vi "trim_string_of_wspaces_and_quotes.vi"(3 "Trim whitespaces (Trim both)":u16(ring) items=["Trim both", "Trim start", "Trim end", "Trim none"], 4 "String in":string, 5 "Remove quotes (Remove All)":u16(ring) items=["Remove All Quotes", "Remove Single Quotes", "Remove Double Quotes", "Remove None"]) -> (1 "String out":string)   [LabVIEW 2020, in "Rohde&Schwarz RTx Oscilloscopes.lvlib" / "rsidr_core.lvlib"]
uses:
  rsidr_core.lvlib
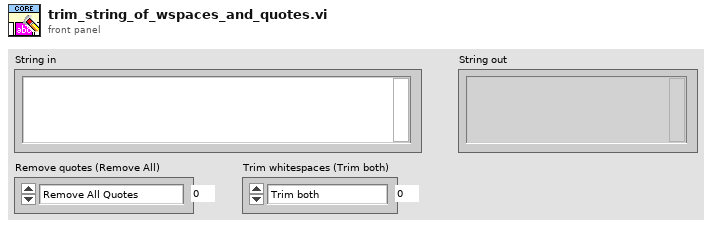
[diagram p1: front panel]
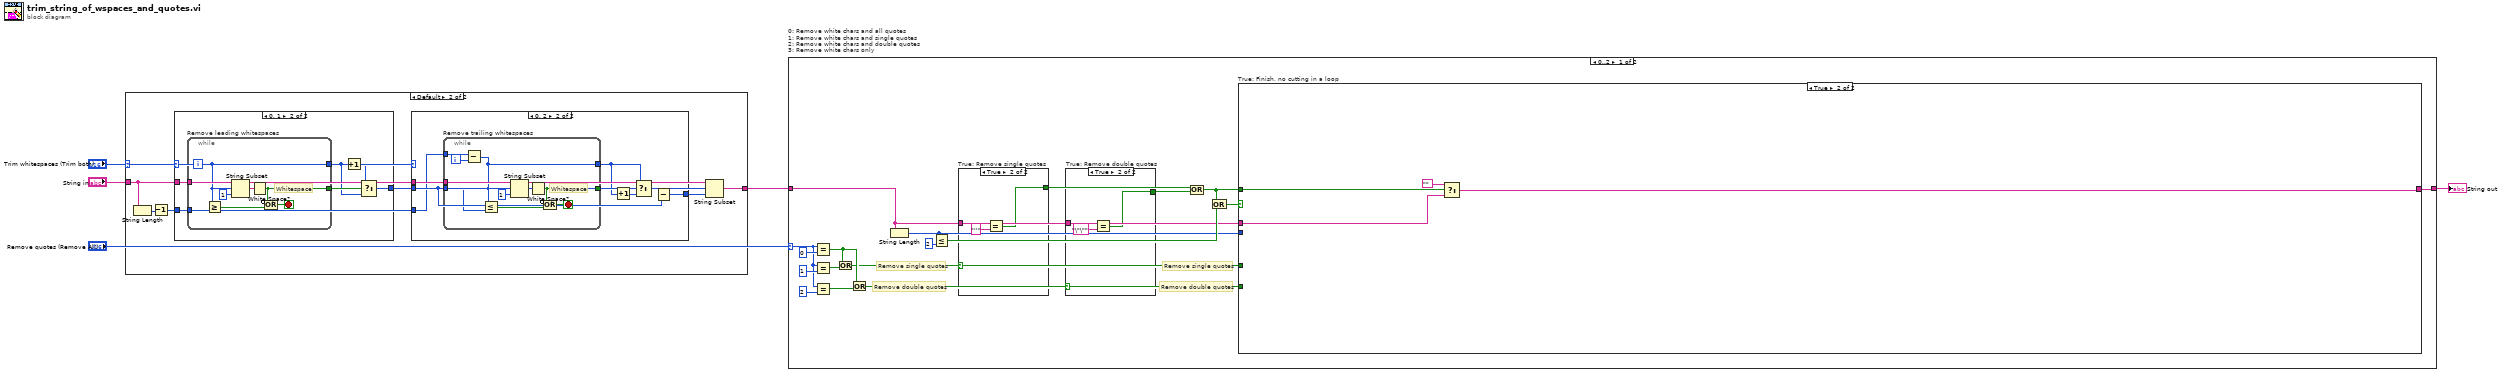
[diagram p0: block diagram]
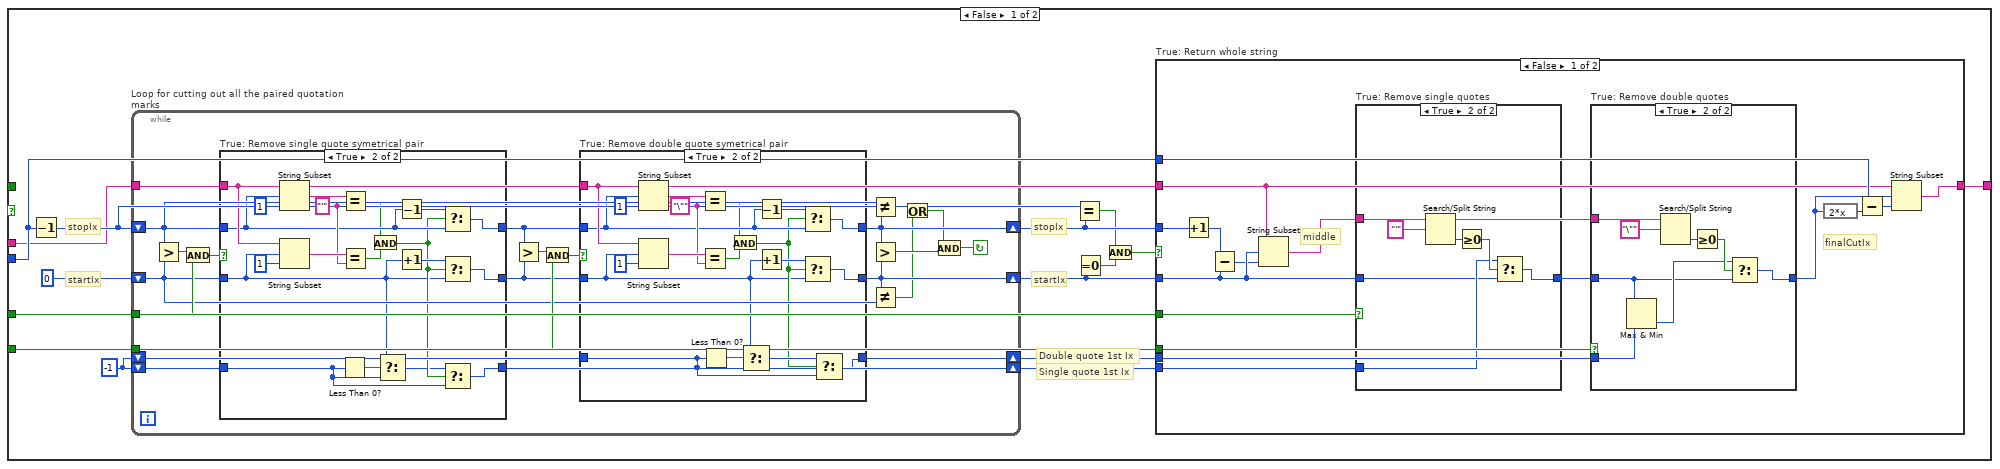
[diagram p5: hidden frame]
diagram:
  n1 = case shown="Default" "Trim whitespaces (Trim both)" {
    selector: "Trim whitespaces (Trim both)" -> [_ w8]
    tunnel: "String in" -> [w6 w13]
    tunnel: [w6 w12] -> w2
    frame 3 {
    }
    frame Default {
      n2 = String Length(string=w13) -> (length=w10:i32)
      n3 = Decrement(x=w10) -> (x-1=w11:i32)
      n4 = case shown="0, 1" w8 {
        tunnel: w13 -> [_ w38]
        tunnel: w11 -> [_ w35]
        tunnel: [_ w34] -> w7
        frame Default {
        }
        frame 0, 1 {
          n5 = while "Remove leading whitespaces" {
            tunnel: w35 -> [w44]
            tunnel: [w41] -> w33
            tunnel: [w39] -> w37
            tunnel: w38 -> [w40]
            i -> [w41]
            stop <- w42 stop-if-true
            # "Whitespace"
            n6 = Greater Or Equal?(x=w41, y=w44) -> (x >= y?=w43:bool)
            n7 = String Subset(string=w40, offset (0)=w41, length (rest)=1 ("length (rest)")) -> (substring=w45:string)
            n8 = White Space?(1:w45) -> (0:w39:bool)
            n9 = Compound Arithmetic op=OR(invert w39, w43) -> (w42:bool)
          }
          n10 = Increment(x=w33) -> (x+1=w36:i32)
          n11 = Select(t=w36, s=w37, f=w33) -> (s? t:f=w34:i32)
        }
      }
      n12 = case shown="0, 2" w8 {
        tunnel: w13 -> [_ w22]
        tunnel: w11 -> [w14 w21]
        tunnel: [w14 w19] -> w9
        tunnel: w7 -> [_ w15]
        frame Default {
        }
        frame 0, 2 {
          n13 = while "Remove trailing whitespaces" {
            tunnel: [w26] -> w17
            tunnel: [w23] -> w20
            tunnel: w22 -> [w29]
            tunnel: w21 -> [w28]
            tunnel: w15 -> [w25]
            i -> [w27]
            stop <- w30 stop-if-true
            # "Whitespace"
            n14 = Subtract(x=w28, y=w27) -> (x-y=w26:i32)
            n15 = Less Or Equal?(x=w26, y=w25) -> (x <= y?=w24:bool)
            n16 = String Subset(string=w29, offset (0)=w26, length (rest)=1 ("length (rest)")) -> (substring=w31:string)
            n17 = White Space?(1:w31) -> (0:w23:bool)
            n18 = Compound Arithmetic op=OR(invert w23, w24) -> (w30:bool)
          }
          n19 = Increment(x=w17) -> (x+1=w18:i32)
          n20 = Select(t=w17, s=w20, f=w18) -> (s? t:f=w16:i32)
          n21 = Subtract(x=w16, y=w15) -> (x-y=w19:i32)
        }
      }
      n22 = String Subset(string=w13, offset (0)=w7, length (rest)=w9) -> (substring=w12:string)
    }
  }
  n23 = case "0: Remove white chars and all quotes\n1: Remove white chars and single quotes\n2: Remove white chars and double quotes\n3: Remove white chars only" shown="0..2" "Remove quotes (Remove All)" {
    selector: "Remove quotes (Remove All)" -> [w61 _]
    tunnel: w2 -> [w47 w190]
    tunnel: [w52 w190] -> w4
    frame 0..2 {
      # "Remove double quotes"
      # "Remove single quotes"
      # "Remove double quotes"
      # "Remove single quotes"
      n24 = Equal?(x=w61, y=u16 0 ("Remove quotes (Remove All)")) -> (x = y?=w58:bool)
      n25 = Equal?(x=w61, y=u16 1) -> (x = y?=w60:bool)
      n26 = Equal?(x=w61, y=u16 2) -> (x = y?=w59:bool)
      n27 = Or(x=w58, y=w60) -> (x .or. y?=w49:bool)
      n28 = Or(x=w58, y=w59) -> (x .or. y?=w48:bool)
      n29 = String Length(string=w47) -> (length=w50:i32)
      n30 = Less Or Equal?(x=w50, y=2) -> (x <= y?=w51:bool)
      n31 = case "True: Remove single quotes" shown="True" w49 {
        tunnel: w47 -> [_ w188]
        tunnel: [_ w187] -> w56
        frame False {
        }
        frame True {
          n32 = Equal?(x=w188, y="''") -> (x = y?=w187:bool)
        }
      }
      n33 = case "True: Remove double quotes" shown="True" w48 {
        tunnel: w47 -> [_ w185]
        tunnel: [_ w184] -> w55
        frame False {
        }
        frame True {
          n34 = Equal?(x=w185, y="\"\"") -> (x = y?=w184:bool)
        }
      }
      n35 = Compound Arithmetic op=OR(w56, w55) -> (w53:bool)
      n36 = Compound Arithmetic op=OR(w53, w51) -> (w54:bool)
      n37 = case "True: Finish, no cutting in a loop" shown="True" w54 {
        tunnel: w47 -> [w65 w182]
        tunnel: w53 -> [_ w183]
        tunnel: [w77 w180] -> w52
        tunnel: w50 -> [w76 _]
        tunnel: w49 -> [w75 _]
        tunnel: w48 -> [w69 _]
        frame False {
          w68 = -1
          # "Double quote 1st Ix"
          # "Single quote 1st Ix"
          # "stopIx"
          # "startIx"
          # "startIx"
          # "stopIx"
          n38 = Decrement(x=w76) -> (x-1=w72:i32)
          n39 = while "Loop for cutting out all the paired quotation marks" {
            shift-right: [w124] -> w71
            shift-left: w72 -> [w123]
            tunnel: w65 -> [w127]
            tunnel: w75 -> [w134]
            tunnel: w69 -> [w130]
            shift-right: [w125] -> w78
            shift-left: 0 -> [w126]
            shift-right: [w116] -> w67
            shift-left: w68 -> [w117]
            shift-right: [w114] -> w66
            shift-left: w68 -> [w115]
            stop <- w121 continue-if-true
            n40 = Greater?(x=w123, y=w126) -> (0:w135:bool)
            n41 = And(x=w135, y=w134) -> (x .and. y?=w133:bool)
            n42 = case "True: Remove single quote symetrical pair" shown="True" w133 {
              tunnel: w127 -> [_ w177]
              tunnel: w126 -> [w159 w162]
              tunnel: w123 -> [w160 w172]
              tunnel: [w160 w171] -> w131
              tunnel: [w159 w170] -> w129
              tunnel: w117 -> [w158 w161]
              tunnel: [w158 w163] -> w116
              frame False {
              }
              frame True {
                w174 = "'" ("y")
                n43 = String Subset(string=w177, offset (0)=w172, length (rest)=1 ("length (rest)")) -> (substring=w176:string)
                n44 = String Subset(string=w177, offset (0)=w162, length (rest)=1 ("length (rest)")) -> (substring=w175:string)
                n45 = Less Than 0?(x=w161) -> (x < 0?=w165:bool)
                n46 = Equal?(x=w176, y=w174) -> (x = y?=w168:bool)
                n47 = Equal?(x=w175, y=w174) -> (x = y?=w167:bool)
                n48 = And(x=w168, y=w167) -> (x .and. y?=w166:bool)
                n49 = Select(t=w162, s=w165, f=w161) -> (s? t:f=w164:i32)
                n50 = Decrement(x=w172) -> (x-1=w173:i32)
                n51 = Increment(x=w162) -> (x+1=w169:i32)
                n52 = Select(t=w173, s=w166, f=w172) -> (s? t:f=w171:i32)
                n53 = Select(t=w169, s=w166, f=w162) -> (s? t:f=w170:i32)
                n54 = Select(t=w164, s=w166, f=w161) -> (s? t:f=w163:i32)
              }
            }
            n55 = Greater?(x=w131, y=w129) -> (0:w132:bool)
            n56 = And(x=w132, y=w130) -> (x .and. y?=w128:bool)
            n57 = case "True: Remove double quote symetrical pair" shown="True" w128 {
              tunnel: w127 -> [_ w155]
              tunnel: w129 -> [w137 w139]
              tunnel: w131 -> [w138 w150]
              tunnel: [w138 w149] -> w124
              tunnel: [w137 w148] -> w125
              tunnel: w115 -> [w136 w142]
              tunnel: [w136 w141] -> w114
              frame False {
              }
              frame True {
                w152 = "\"" ("y")
                n58 = String Subset(string=w155, offset (0)=w150, length (rest)=1 ("length (rest)")) -> (substring=w154:string)
                n59 = String Subset(string=w155, offset (0)=w139, length (rest)=1 ("length (rest)")) -> (substring=w153:string)
                n60 = Equal?(x=w154, y=w152) -> (x = y?=w146:bool)
                n61 = Equal?(x=w153, y=w152) -> (x = y?=w145:bool)
                n62 = Less Than 0?(x=w142) -> (x < 0?=w143:bool)
                n63 = And(x=w146, y=w145) -> (x .and. y?=w140:bool)
                n64 = Select(t=w139, s=w143, f=w142) -> (s? t:f=w144:i32)
                n65 = Decrement(x=w150) -> (x-1=w151:i32)
                n66 = Increment(x=w139) -> (x+1=w147:i32)
                n67 = Select(t=w151, s=w140, f=w150) -> (s? t:f=w149:i32)
                n68 = Select(t=w147, s=w140, f=w139) -> (s? t:f=w148:i32)
                n69 = Select(t=w144, s=w140, f=w142) -> (s? t:f=w141:i32)
              }
            }
            n70 = Not Equal?(x=w123, y=w124) -> (x != y?=w120:bool)
            n71 = Greater?(x=w124, y=w125) -> (0:w122:bool)
            n72 = Not Equal?(x=w125, y=w126) -> (x != y?=w119:bool)
            n73 = Or(x=w120, y=w119) -> (x .or. y?=w118:bool)
            n74 = Compound Arithmetic op=AND(w118, w122) -> (w121:bool)
          }
          n75 = Equal?(x=w72, y=w71) -> (x = y?=w70:bool)
          n76 = Equal To 0?(x=w78) -> (x = 0?=w73:bool)
          n77 = And(x=w70, y=w73) -> (x .and. y?=w74:bool)
          n78 = case "True: Return whole string" shown="False" w74 {
            tunnel: w78 -> [w81 _]
            tunnel: [w92 w113] -> w77
            tunnel: w76 -> [w93 _]
            tunnel: w75 -> [w90 _]
            tunnel: w71 -> [w91 _]
            tunnel: w69 -> [w85 _]
            tunnel: w67 -> [w88 _]
            tunnel: w66 -> [w86 _]
            tunnel: w65 -> [w82 w113]
            frame False {
              # "middle"
              # "finalCutIx"
              n79 = Increment(x=w91) -> (x+1=w89:i32)
              n80 = Subtract(x=w89, y=w81) -> (x-y=w80:i32)
              n81 = String Subset(string=w82, offset (0)=w81, length (rest)=w80) -> (substring=w83:string)
              n82 = case "True: Remove single quotes" shown="True" w90 {
                tunnel: [w105 w107] -> w87
                tunnel: w81 -> [w105 w106]
                tunnel: w83 -> [_ w112]
                tunnel: w88 -> [_ w108]
                frame False {
                }
                frame True {
                  n83 = Search/Split String(string=w112, search string/char (-)="'" ("y")) -> (offset of match=w110:i32)  [unwired: 1 in, 2 out]
                  n84 = Greater Or Equal To 0?(x=w110) -> (x >= 0?=w109:bool)
                  n85 = Select(t=w108, s=w109, f=w106) -> (s? t:f=w107:i32)
                }
              }
              n86 = case "True: Remove double quotes" shown="True" w85 {
                tunnel: [w96 w100] -> w84
                tunnel: w83 -> [_ w104]
                tunnel: w87 -> [w96 w97]
                tunnel: w86 -> [_ w99]
                frame False {
                }
                frame True {
                  n87 = Max & Min(x=w97, y=w99) -> (min(x,y)=w98:i32)  [unwired: 1 out]
                  n88 = Search/Split String(string=w104, search string/char (-)="\"" ("y")) -> (offset of match=w102:i32)  [unwired: 1 in, 2 out]
                  n89 = Greater Or Equal To 0?(x=w102) -> (x >= 0?=w101:bool)
                  n90 = Select(t=w98, s=w101, f=w97) -> (s? t:f=w100:i32)
                }
              }
              n91 = expression code="2*x"(w84) -> (w95:i32)
              n92 = Subtract(x=w93, y=w95) -> (x-y=w94:i32)
              n93 = String Subset(string=w82, offset (0)=w84, length (rest)=w94) -> (substring=w92:string)
            }
            frame True {
            }
          }
        }
        frame True {
          n94 = Select(t="" ("Empty String Constant"), s=w183, f=w182) -> (s? t:f=w180:string)
        }
      }
    }
    frame 3, Default {
    }
  }
  "String out" <- w4
